vi "read csv.vi"(8 "error in (no error)":errorcluster, 10 "String":string, 11 "Path":path) -> (0 "error out":errorcluster)   [LabVIEW 2019]
uses:
  Write Mode.ctl
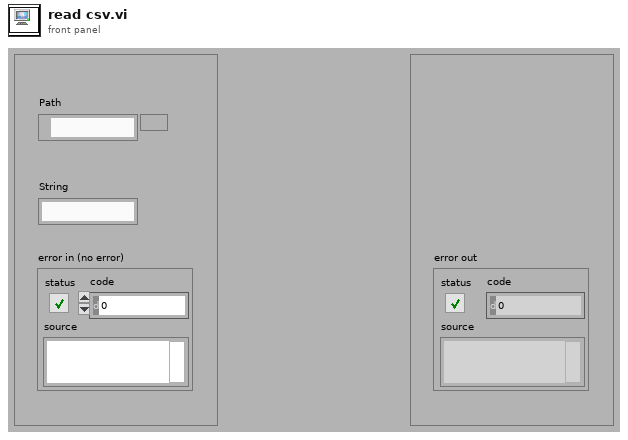
[diagram p1: front panel]
types:
  T1 = typedef "Write Mode.ctl" = enum16{"GetRef", "Initialize", "Close"}
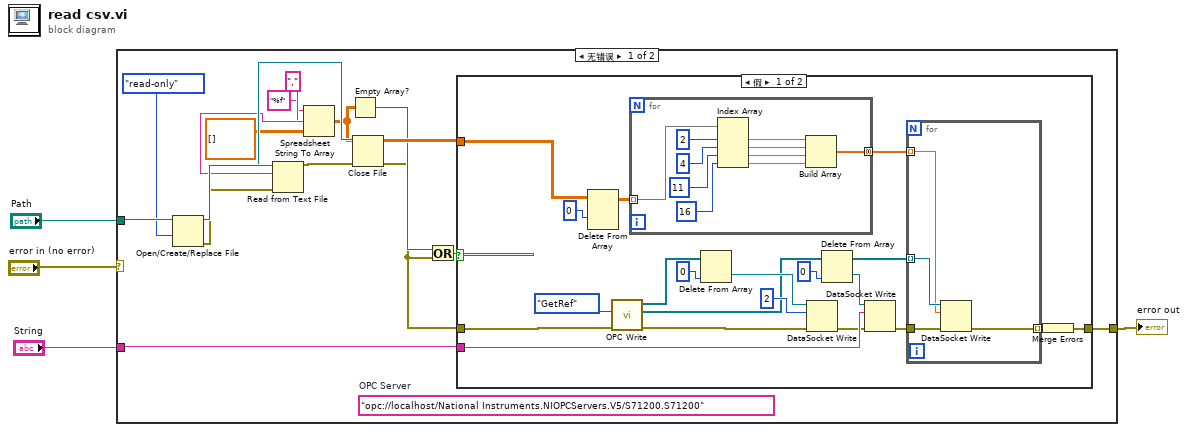
[diagram p0: block diagram]
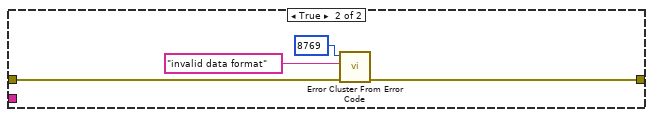
[diagram p2: hidden frame]
diagram:
  n1 = case shown="无错误" "error in (no error)" {
    selector: "error in (no error)" -> [_ w59]
    tunnel: "Path" -> [w20 _]
    tunnel: "String" -> [w10 _]
    tunnel: [w9 w59] -> w2
    frame No Error {
      (unwired) "opc://localhost/National Instruments.NIOPCServers.V5/S71200.S71200"  # OPC Server
      n2 = Open/Create/Replace File(file path (use dialog)=w20, access (0:read/write)=enum16{"read/write", "read-only", "write-only"}."read-only") -> (refnum out=w18:refnum<file>, error out=w17:errorcluster)  [unwired: 4 in, 1 out]
      n3 = Read from Text File(file (use dialog)=w18, error in=w17) -> (refnum out=w16:refnum<file>, text=w14:string, error out=w15:errorcluster)  [unwired: 2 in, 1 out]
      n4 = Spreadsheet String To Array(delimiter (Tab)=",", format string="%f", spreadsheet string=w14, array type (2D Dbl)=dbl[][] []) -> (array=w8:dbl[][])
      n5 = Empty Array?(array=w8) -> (empty?=w7:bool)
      n6 = Close File(refnum=w16, error in=w15) -> (error out=w5:errorcluster)  [unwired: 1 out]
      n7 = Or(x=w7, y=w5) -> (x .or. y?=w6:bool)
      n8 = case shown="假" w6 {
        tunnel: w10 -> [w30 _]
        tunnel: [w36 w57] -> w9
        tunnel: w8 -> [w34 _]
        tunnel: w5 -> [w23 w58]
        frame False {
          n9 = Delete From Array(array=w34, index (row)=0) -> (array with subset deleted=w39:dbl[][])  [unwired: 2 in, 1 out]
          n10 = call "OPC Write.vi"("error in (no error)"=w23, "Mode"=Write_Mode."GetRef") -> ("error out"=w22:errorcluster, "data ref"=w21:refnum<k13>[], "all ref"=w27:refnum<k13>[])  [unwired: 7 in]
          n11 = for {
            tunnel: w39 -> [w54] mode=indexing
            tunnel: [w49] -> w38 mode=concatenating
            n12 = Index Array(array=w54, index #1=2 ("index"), index #2=4 ("index"), index #3=11 ("index"), index #4=16 ("index")) -> (element #1=w52:dbl, element #2=w53:dbl, element #3=w51:dbl, element #4=w50:dbl)
            n13 = Build Array(w52, w53, w51, w50) -> (w49:dbl[])
          }
          n14 = Delete From Array(array=w27, index=0) -> (deleted portion=w25:refnum<k13>)  [unwired: 1 in, 1 out]
          n15 = DataSocket Write(8:w22, 10:2, 11:w25) -> (0:w28:errorcluster)  [unwired: 1 in, 2 out]
          n16 = Delete From Array(array=w21, index=0) -> (deleted portion=w33:refnum<k13>, array with subset deleted=w31:refnum<k13>[])  [unwired: 1 in]
          n17 = DataSocket Write(8:w28, 10:w30, 11:w33) -> (0:w32:errorcluster)  [unwired: 1 in, 2 out]
          n18 = for {
            tunnel: w31 -> [w44] mode=indexing
            tunnel: w32 -> [w43]
            tunnel: w38 -> [w42] mode=indexing
            tunnel: [w41] -> w37 mode=indexing
            n19 = DataSocket Write(8:w43, 10:w42, 11:w44) -> (0:w41:errorcluster)  [unwired: 1 in, 2 out]
          }
          n20 = Merge Errors(w37) -> (w36:errorcluster)
        }
        frame True {
          n21 = call <vilib>:"Error Cluster From Error Code.vi"("error in (no error)"=w58, "error message (\"\")"="invalid data format" ("error message (\"\")"), "error code (0)"=8769) -> ("error out"=w57:errorcluster)  [unwired: 6 in]
        }
      }
    }
    frame Error {
    }
  }
  "error out" <- w2
